vi "CreateTextureFromSurface.vi"(8 "No Error":errorcluster, 10 "Surface [SDL_Surface *]":i64 format="%.0x", 11 "Renderer [SDL_Renderer *]":i64 format="%.0x") -> (0 "error out":errorcluster, 3 "Texture [SDL_Texture *]":i64 format="%.0x")   [LabVIEW 2024, in "SDL3.lvlib" / "Render.lvlib"]
doc: "<B>Summary</B>\nCreate a texture from an existing surface.\n\n<B>Remarks</B>\nThe surface is not modified or freed by this function.\n\nThe SDL_TextureAccess hint for the created texture is <B>SDL_TEXTUREACCESS_STATIC</B>.\n\nThe pixel format of the created texture may be different from the pixel format of the surface, and can be queried using the <B>SDL_PROP_TEXTURE_FORMAT_NUMBER</B> property."
uses:
  <vilib>/Utility/error.llb/Error Cluster From Error Code.vi
  Render.lvlib
  Error/Error.lvlib
  Lib/Win32/SDL3.dll
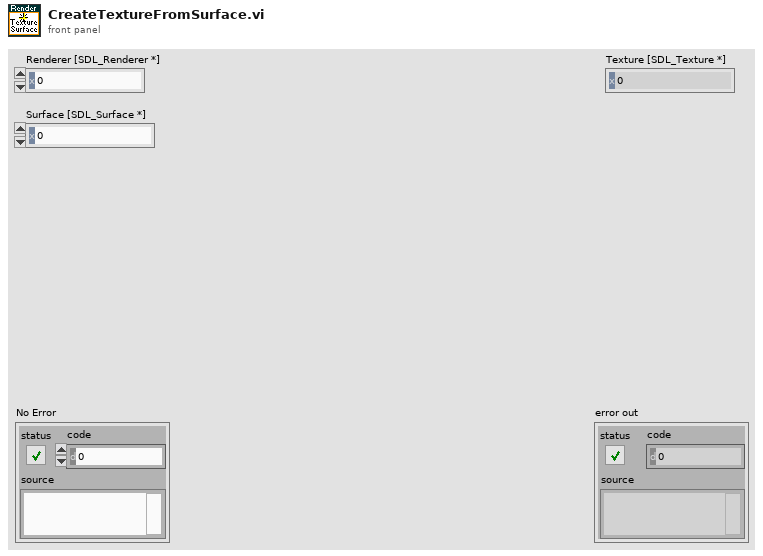
[diagram p1: front panel]
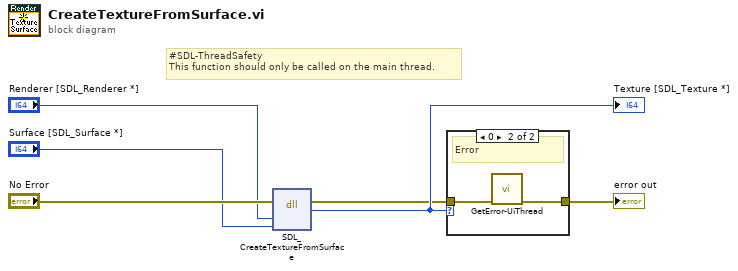
[diagram p0: block diagram]
diagram:
  # "#SDL-ThreadSafety\nThis function should only be called on the main thread."
  n1 = dll-call lib="C:/Users/Thomas/Documents/Projects/LV-SDL3/Lib/Win32/SDL3.dll" fn="SDL_CreateTextureFromSurface" label="SDL3-*.*:SDL_CreateTexture"(error in="No Error", "renderer"="Renderer [SDL_Renderer *]", "surface"="Surface [SDL_Surface *]") -> (error out=w2:errorcluster, "return type"=w4:i64)  [unwired: 4 in, 1 out]
  "Texture [SDL_Texture *]" <- w4
  n2 = case shown="0" w4 {
    tunnel: w2 -> [w7 w9]
    tunnel: [w7 w8] -> w5
    frame Default {
      # "Ok"
    }
    frame 0 {
      # "Error"
      n3 = call "GetError-UiThread.vi"("No Error"=w9) -> ("error out"=w8:errorcluster)  [unwired: 10 in]
    }
  }
  "error out" <- w5
